vi "find_head_angle.vi"(6 "Numeric":i32, 9 "Numeric 2":i32, 10 "Numeric 3":i32, 11 "Centerline":dbl[][](array[numeric])) -> (3 "Numeric 4":dbl)   [LabVIEW 2019]
uses:
  <vilib>/Analysis/baseanly.llb/Real Dot Product.vi
  <vilib>/Analysis/_algsub.llb/Real Vector Norm.vi
  <vilib>/Analysis/NI_AALPro.lvlib
  <vilib>/Analysis/NI_AALBase.lvlib
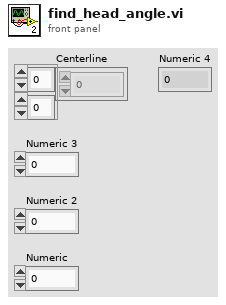
[diagram p1: front panel]
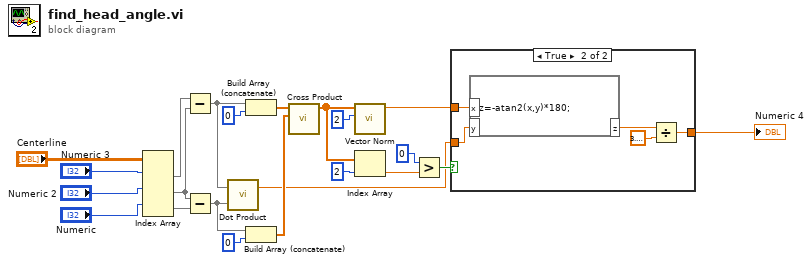
[diagram p0: block diagram]
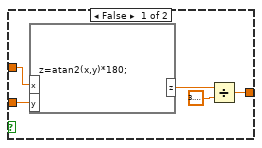
[diagram p2: hidden frame]
diagram:
  n1 = Index Array(array="Centerline", index (row) #1="Numeric 3", index (row) #2="Numeric 2", index (row) #3="Numeric") -> (element #1=w14:dbl[], element #2=w13:dbl[], element #3=w12:dbl[])  [unwired: 3 in]
  n2 = Subtract(x=w14, y=w13) -> (x-y=w5:dbl[])
  n3 = Subtract(x=w13, y=w12) -> (x-y=w4:dbl[])
  n4 = call-poly <vilib>:"Dot Product.vi"("Y Vector"=w4, "X Vector"=w5) -> ("X * Y"=w3:dbl)  [unwired: 1 out]
  n5 = Build Array (concatenate)(w5, 0) -> (w19:dbl[])
  n6 = Build Array (concatenate)(w4, 0) -> (w18:dbl[])
  n7 = call <vilib>:"Cross Product.vi"("B Vector"=w18, "A Vector"=w19) -> ("Cross Product"=w8:dbl[])  [unwired: 8 in, 1 out]
  n8 = call-poly <vilib>:"Vector Norm.vi"("norm type"=2, "Input Vector"=w8) -> ("norm"=w6:dbl)  [unwired: 8 in, 1 out]
  n9 = Index Array(array=w8, index=2) -> (element=w1:dbl)
  n10 = Greater?(x=0, y=w1) -> (0:w11:bool)
  n11 = case shown="True" w11 {
    tunnel: w6 -> [w27 w32]
    tunnel: w3 -> [w26 w31]
    tunnel: [w23 w28] -> w2
    frame False {
      n12 = formula code="z=atan2(x,y)*180;"("x"=w27, "y"=w26) -> ("z"=w24:dbl)
      n13 = Divide(x=w24, y=3.141592653589793) -> (x/y=w23:dbl)
    }
    frame True {
      n14 = formula code="z=-atan2(x,y)*180;"("x"=w32, "y"=w31) -> ("z"=w29:dbl)
      n15 = Divide(x=w29, y=3.141592653589793) -> (x/y=w28:dbl)
    }
  }
  "Numeric 4" <- w2
